vi "Introspection Core.vi"(8 "error in (no error)":errorcluster, 11 "BNT_DAQmx-MCSV-DOPWM in":refnum<class "BNT_DAQmx-MCSV-DOPWM.lvclass">) -> (0 "error out":errorcluster, 2 "CSPPMessages":refnum<class "Message.lvclass">[](array[class]), 3 "BNT_DAQmx-MCSV-DOPWM out":refnum<class "BNT_DAQmx-MCSV-DOPWM.lvclass">)   [LabVIEW 2019, in "BNT_DAQmx.lvlib" / "BNT_DAQmx-MCSV-DOPWM.lvclass"]
doc: "This vi delivers a list with all messages this actor reacts to. \n\nNote that all inherited classes have to overwrite it."
uses:
  BNT_DAQmx-MCSV-DOPWM.lvclass
  <vilib>/ActorFramework/Message/Message.lvclass
  BNT_DAQmx-MCSV-DOPWM Messages/Set Ratio Msg/Set Ratio Msg.lvclass
  C:/Program Files (x86)/National Instruments/LabVIEW 2019/vi.lib/ActorFramework/Message/Message.lvclass
  BNT_DAQmx-MCSV-DOPWM Messages/Set Ratios Msg/Set Ratios Msg.lvclass
  BNT_DAQmx-MCSV-DOPWM Messages/Set Delay Msg/Set Delay Msg.lvclass
  BNT_DAQmx-MCSV-DOPWM Messages/Set Delays Msg/Set Delays Msg.lvclass
  BNT_DAQmx-MCSV-DOPWM Messages/Set Length Msg/Set Length Msg.lvclass
  BNT_DAQmx-MCSV-DOPWM Messages/Set Lengths Msg/Set Lengths Msg.lvclass
  BNT_DAQmx-MCSV/BNT_DAQmx-MCSV.lvclass
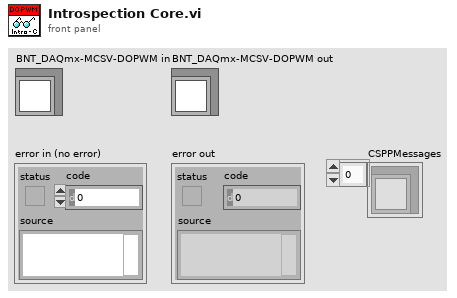
[diagram p1: front panel]
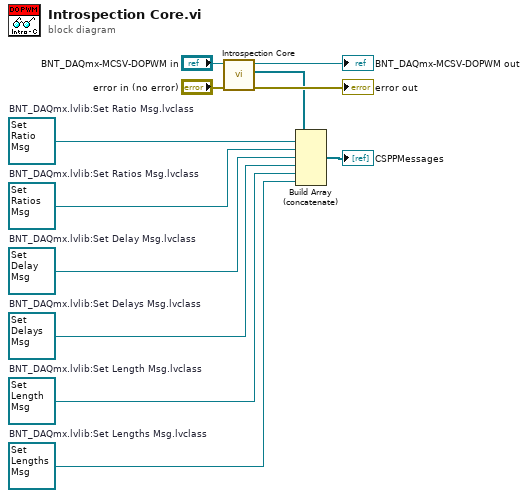
[diagram p0: block diagram]
diagram:
  w1 = refnum<class "Set Lengths Msg.lvclass"> refnum  # BNT_DAQmx.lvlib:Set Lengths Msg.lvclass
  w2 = refnum<class "Set Length Msg.lvclass"> refnum  # BNT_DAQmx.lvlib:Set Length Msg.lvclass
  w3 = refnum<class "Set Delays Msg.lvclass"> refnum  # BNT_DAQmx.lvlib:Set Delays Msg.lvclass
  w4 = refnum<class "Set Delay Msg.lvclass"> refnum  # BNT_DAQmx.lvlib:Set Delay Msg.lvclass
  w5 = refnum<class "Set Ratios Msg.lvclass"> refnum  # BNT_DAQmx.lvlib:Set Ratios Msg.lvclass
  w6 = refnum<class "Set Ratio Msg.lvclass"> refnum  # BNT_DAQmx.lvlib:Set Ratio Msg.lvclass
  n1 = call-parent "Introspection Core.vi"("error in (no error)"="error in (no error)", "BNT_DAQmx-MCSV in"="BNT_DAQmx-MCSV-DOPWM in") -> ("error out"=→"error out":errorcluster, "CSPPMessages"=w11:refnum<class "Message.lvclass">[], "BNT_DAQmx-MCSV out"=→"BNT_DAQmx-MCSV-DOPWM out":refnum<class "BNT_DAQmx-MCSV-DOPWM.lvclass">)  [unwired: 7 in]
  n2 = Build Array (concatenate)(w11, w6, w5, w4, w3, w2, w1) -> (→"CSPPMessages":refnum<class "Message.lvclass">[])
